vi "JAS-Color Sensor V3 Add Color Match.vi"(10 "Color":cluster{"R":dbl, "G":dbl, "B":dbl}, 11 "Name":string) -> (3 "ColorIndex":i32)   [LabVIEW 2019]
uses:
  <vilib>/Rock Robotics/WPI/ThirdParty/REV Robotics/Color SensorV3/Typedef/Color Sensor V3 Color Match.ctl
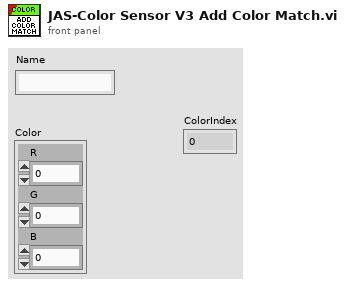
[diagram p1: front panel]
types:
  T1 = typedef "Color Sensor V3 Color Match.ctl" = cluster{"Name":string, "Normalized Color":cluster{"R":dbl, "G":dbl, "B":dbl}}
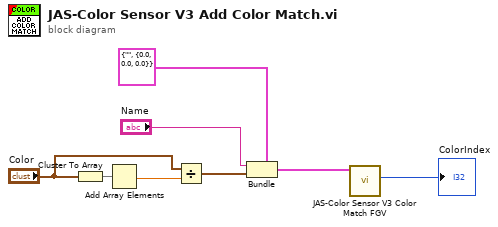
[diagram p0: block diagram]
diagram:
  n1 = Cluster To Array(cluster="Color") -> (array=w5:dbl[])
  n2 = Add Array Elements(numeric array=w5) -> (sum=w4:dbl)
  n3 = Divide(x="Color", y=w4) -> (x/y=w2:cluster{"R":dbl, "G":dbl, "B":dbl})
  n4 = Bundle(cluster=T1 {"Name"="", "Normalized Color"={"R"=0.0, "G"=0.0, "B"=0.0}} ("output cluster"), "Name"="Name", "Normalized Color"=w2) -> (w6:T1)
  n5 = call "JAS-Color Sensor V3 Color Match FGV.vi"("Color Match"=w6) -> ("LastIndex"=→"ColorIndex":i32)  [unwired: 9 in, 1 out]
